vi "Test_Benchmarking_LocalLogEventCall_AvgCallTimeSub10uS.vi"(8 "error in (no error)":errorcluster, 11 "Benchmarking in":refnum<class "Benchmarking.lvclass">) -> (0 "error out":errorcluster, 3 "Benchmarking out":refnum<class "Benchmarking.lvclass">)   [LabVIEW 2017, in "Benchmarking.lvclass"]
uses:
  Benchmarking.lvclass
  Source/Composed Log/LoggerReference/LoggerReference.lvclass/LoggerReference.ctl
  Source/Composed Log/Types/Log Level.ctl
  c732dfe6-6ae6-40e1-b7d0-4452a78b430e.vi
  <vilib>/Analysis/baseanly.llb/Mean (DBL).vi
  Source/Composed Log/LoggerReference/Return Aggregate Queues.vi
  Source/Composed Log/LoggerReference/Add Aggregate Log.vi
  c732dfe6-6ae6-40e1-b7d0-4452a78b430e.vi/b90949e6-ac07-4381-bf2f-417c398e7aa0.vi
  Source/Composed Log/LoggerReference/Log.vi
  Source/Composed Log/LoggerReference/Get Valid Event Time.vi
  Source/Composed Log/LoggerReference/Send Add Sink.vi
  Source/Composed Log/LoggerReference/Remove Stale Logs.vi
  Source/LVQueue Sink/LVQueue Sink.lvclass
  C:/CS/Internal/LabVIEW/Logger/Source/Composed Log/Log Sink/Log Sink.lvclass
  Source/Composed Log/Application Logger/Launch Worker Loop.vi
  Source/Composed Log/LoggerReference/Initialize Logger Instance.vi
  Source/Composed Log/LoggerReference/LoggerReference.lvclass
  Source/Composed Log/IErrorFormat/IErrorFormat.lvclass
  Source/Composed Log/Log Sink/Log Sink.lvclass
  Source/Composed Log/Composed Log.lvlib
  <vilib>/Analysis/NI_AALBase.lvlib
  <vilib>/addons/_JKI Toolkits/VI Tester/TestCase.llb/TestCase.lvclass
  C:/Program Files (x86)/National Instruments/LabVIEW 2017/vi.lib/addons/_JKI Toolkits/VI Tester/TestCase.llb/TestCase.lvclass
panel:
  in  "Numeric":i32=10000
  out "min index(es)":i32
  out "max index(es)":i32
  out "Histogram Graph":T1(graph)
  out "Benchmark Results":string
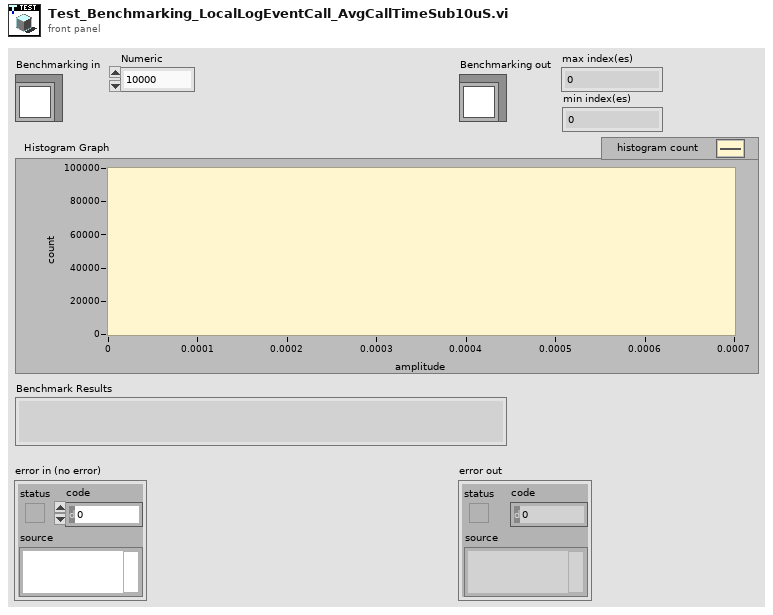
[diagram p1: front panel]
types:
  T1 = cluster{"X Values":dbl[], "Histogram: h(x)":i32[]}
  T2 = typedef "Composed Log.lvlib/Log Level.ctl" = enum16{"Debug", "Info", "Warning", "Error", "Critical"}
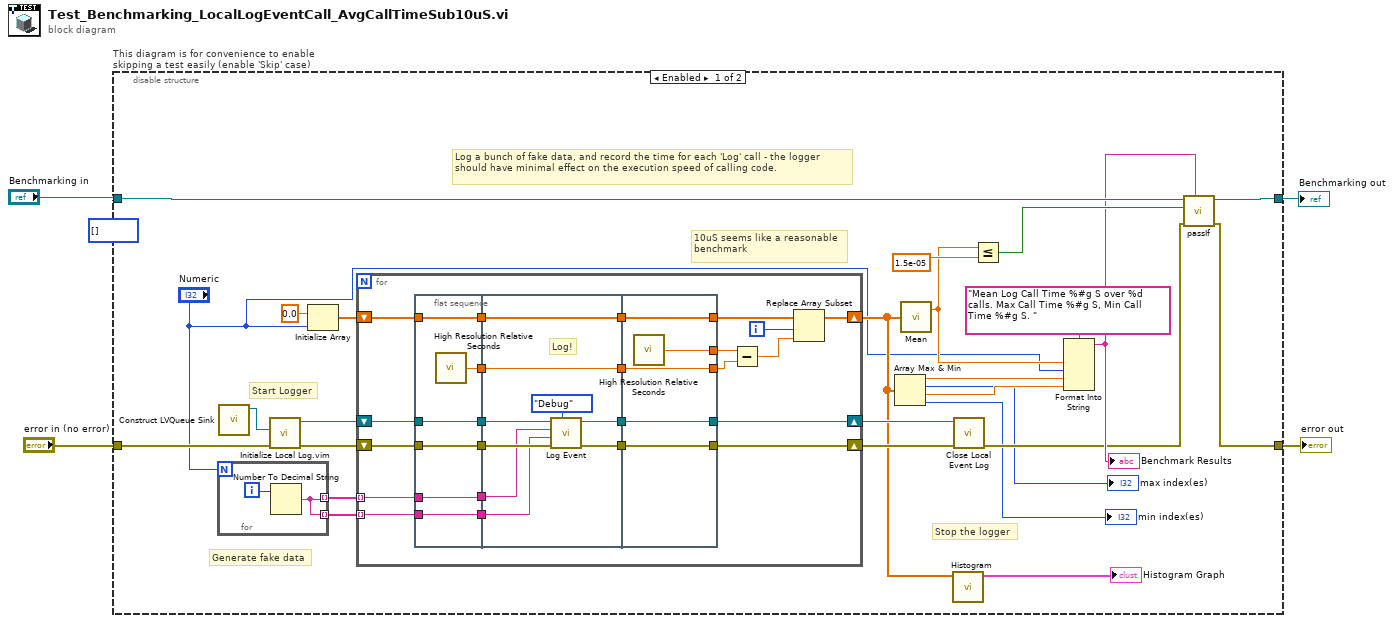
[diagram p0: block diagram]
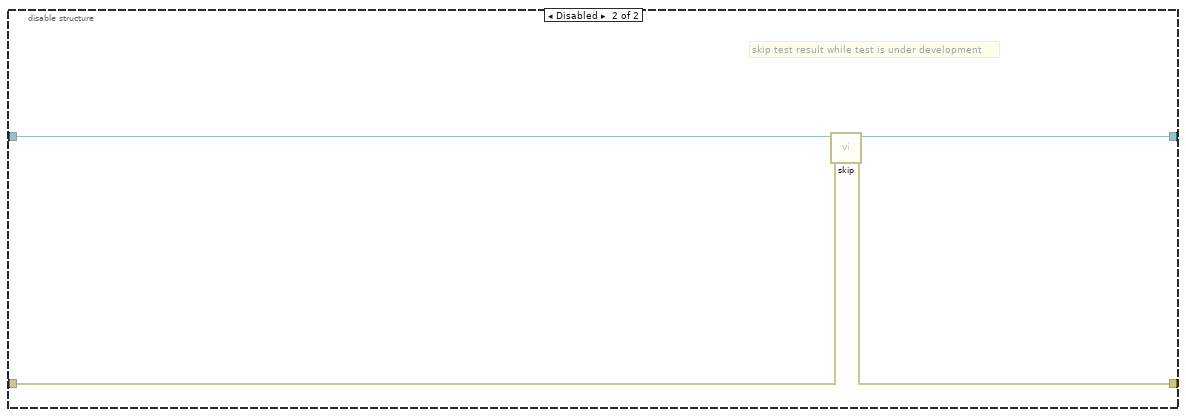
[diagram p2: hidden frame]
diagram:
  n1 = disable-structure "This diagram is for convenience to enable skipping a test easily (enable 'Skip' case)" shown="Enabled" {
    disable-tunnel: "Benchmarking in" -> [w29 w79]
    disable-tunnel: [w28 w77] -> w4
    disable-tunnel: [w30 w78] -> w3
    disable-tunnel: "error in (no error)" -> [w27 w76]
    frame Enabled {
      (unwired) i32[] []
      # "Stop the logger"
      # "10uS seems like a reasonable    benchmark"
      # "Generate fake data"
      # "Start Logger"
      # "Log a bunch of fake data, and record the time for each 'Log' call - the logger should have minimal effect on the execution speed of calling code."
      n2 = for {
        N: "Numeric" -> [_]
        tunnel: [w74] -> w26 mode=indexing
        tunnel: [w74] -> w23 mode=indexing
        i -> [w75]
        n3 = Number To Decimal String(number=w75) -> (decimal integer string=w74:string)  [unwired: 1 in]
      }
      n4 = call "Construct LVQueue Sink.vi"() -> ("LVQueue Sink out"=w13:refnum<class "LVQueue Sink.lvclass">)  [unwired: 10 in, 1 out]
      n5 = call "Initialize Local Log.vim"("error in (no error)"=w27, "Startup Sink(s)"=w13) -> ("error out"=w14:errorcluster, "Log Instance Reference"=w12:refnum<class "LoggerReference.lvclass">)  [unwired: 7 in, 1 out]
      n6 = Initialize Array(0.0 ("element"), "Numeric") -> (w24:dbl[])
      n7 = for {
        tunnel: w26 -> [w48] mode=indexing
        shift-right: [w46] -> w16
        shift-left: w14 -> [w47]
        shift-right: [w37] -> w10
        shift-left: w24 -> [w43]
        tunnel: w23 -> [w36] mode=indexing
        shift-right: [w32] -> w11
        shift-left: w12 -> [w31]
        i -> [w39]
        n8 = flat-sequence {
          tunnel: w47 -> [w58]
          tunnel: w48 -> [w59]
          tunnel: [w59] -> w53
          tunnel: [w58] -> w52
          tunnel: [w57] -> w51
          tunnel: w43 -> [w56]
          tunnel: [w56] -> w41
          tunnel: w36 -> [w55]
          tunnel: [w55] -> w35
          tunnel: [w54] -> w34
          tunnel: w31 -> [w54]
          tunnel: w53 -> [w64]
          tunnel: w52 -> [w68]
          tunnel: w51 -> [w66]
          tunnel: [w67] -> w50
          tunnel: [w66] -> w49
          tunnel: [w65] -> w42
          tunnel: w41 -> [w65]
          tunnel: w35 -> [w63]
          tunnel: w34 -> [w62]
          tunnel: [w61] -> w33
          tunnel: [w72] -> w45
          tunnel: [w73] -> w46
          tunnel: w50 -> [w73]
          tunnel: w49 -> [w72]
          tunnel: [w71] -> w44
          tunnel: [w70] -> w40
          tunnel: w42 -> [w70]
          tunnel: w33 -> [w69]
          tunnel: [w69] -> w32
          frame #0 {
            n9 = call <vilib>:"High Resolution Relative Seconds.vi"() -> ("relative seconds"=w57:dbl)
          }
          frame #1 {
            # "Log!"
            n10 = call "Log Event.vi"("Event Level"=Log_Level."Debug", "error in (no error)"=w68, "Data To Log"=w63, "SourceID"=w64, "Log Instance"=w62) -> ("error out"=w67:errorcluster, "Log Instance Out"=w61:refnum<class "LoggerReference.lvclass">)  [unwired: 5 in]
          }
          frame #2 {
            n11 = call <vilib>:"High Resolution Relative Seconds.vi"() -> ("relative seconds"=w71:dbl)
          }
        }
        n12 = Subtract(x=w44, y=w45) -> (x-y=w38:dbl)
        n13 = Replace Array Subset(array=w40, new element=w38, index=w39) -> (w37:dbl[])
      }
      n14 = Array Max & Min(array=w10) -> (max value=w19:dbl, max index (indices)=→"max index(es)":i32, min value=w18:dbl, min index (indices)=→"min index(es)":i32)
      n15 = call-poly <vilib>:"Mean.vi"("X"=w10) -> ("mean"=w7:dbl)  [unwired: 1 out]
      n16 = call <vilib>:"Histogram.vi"("X"=w10) -> ("Histogram Graph"=→"Histogram Graph":T1)  [unwired: 7 in, 3 out]
      n17 = call "Close Local Event Log.vi"("error in (no error)"=w16, "Log Instance"=w11) -> ("error out"=w15:errorcluster)  [unwired: 9 in]
      n18 = Less Or Equal?(x=w7, y=1.5e-05) -> (x <= y?=w21:bool)
      n19 = Format Into String(format string="Mean Log Call Time %#g S over %d calls. Max Call Time %#g S, Min Call Time %#g S. ", w7, "Numeric", w19, w18) -> (resulting string=w17:string)  [unwired: 2 in, 1 out]
      "Benchmark Results" <- w17
      n20 = call-dynamic "passIf.vi"("custom report message (\"\")"=w17, "error in (no error)"=w15, "pass"=w21, "TestCase in"=w29) -> ("error out"=w30:errorcluster, "TestCase out"=w28:refnum<class "Benchmarking.lvclass">)  [unwired: 6 in]
    }
    frame Disabled {
      # "skip test result while test is under development"
      n21 = call <vilib>:"skip.vi"("error in (no error)"=w76, "TestCase in"=w79) -> ("error out"=w78:errorcluster, "TestCase out"=w77:refnum<class "Benchmarking.lvclass">)  [unwired: 8 in]
    }
  }
  "error out" <- w3
  "Benchmarking out" <- w4
